vi "usrp get clock source.vi"(7 "strbuffer_len":u64, 8 "error in (no error)":errorcluster, 9 "clock_source_out":string, 10 "mboard":u64, 11 "h":u64) -> (0 "error out":errorcluster, 1 "clock_source_out out":string, 3 "function return":u32(ring))   [LabVIEW 2023, in "uhd.lvlib"]
doc: "UHD_API uhd_error uhd_usrp_get_clock_source(\n uhd_usrp_handle h, size_t mboard, char* clock_source_out, size_t strbuffer_len);"
uses:
  <userlib>/uhd/uhd.lvlib
  <userlib>/uhd/uhd.dll
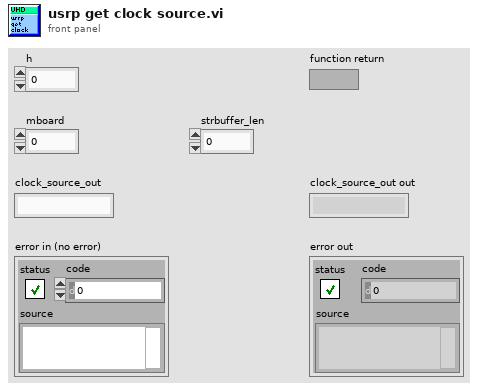
[diagram p1: front panel]
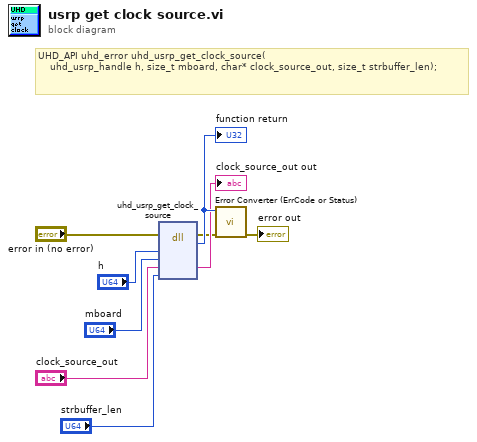
[diagram p0: block diagram]
diagram:
  # "UHD_API uhd_error uhd_usrp_get_clock_source(\n    uhd_usrp_handle h, size_t mboard, char* clock_source_out, size_t strbuffer_len);"
  n1 = dll-call lib="C:/Program Files/National Instruments/LabVIEW 2023/user.lib/uhd/uhd.*" fn="uhd_usrp_get_clock_source"(error in="error in (no error)", "h"="h", "mboard"="mboard", "clock_source_out"="clock_source_out", "strbuffer_len"="strbuffer_len") -> (error out=w2:errorcluster, w9:u32, "clock_source_out"=→"clock_source_out out":string)  [unwired: 5 in, 1 out]
  "function return" <- w9
  n2 = call <userlib>:"Error Converter (ErrCode or Status).vi"("error in (no error)"=w2, "error code"=w9) -> ("error out"=→"error out":errorcluster)  [unwired: 9 in]
